vi "Init.vi"(8 "error in (no error)":errorcluster, 11 "XML Report in":refnum<class "Report.lvclass">) -> (0 "error out":errorcluster, 3 "XML Report out":refnum<class "Report.lvclass">)   [LabVIEW 2020, in "Reports.lvlib" / "Report.lvclass"]
uses:
  Report.lvclass
  C:/git/astemes-lunit/source/Framework/Report Interface/Report Interface.lvclass
  Report.lvclass/Report.ctl
  Report Generator/Report Generator.lvclass
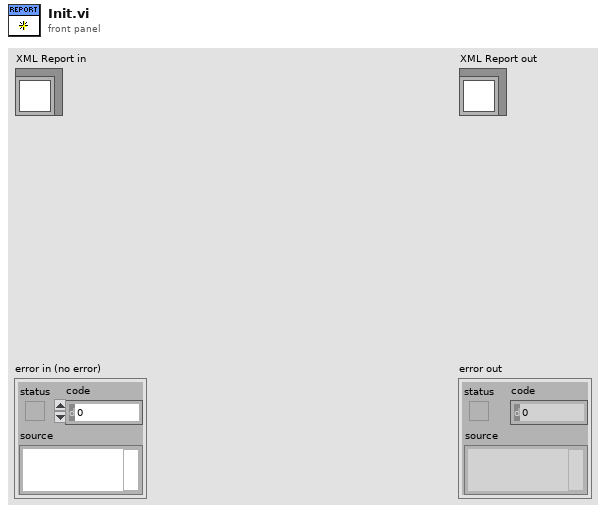
[diagram p1: front panel]
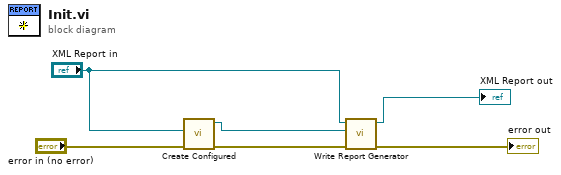
[diagram p0: block diagram]
diagram:
  n1 = call "Create Configured.vi"("error in (no error)"="error in (no error)", "Report Interface"="XML Report in") -> ("error out"=w5:errorcluster, "Report Generator Out"=w2:refnum<class "Report Generator.lvclass">)  [unwired: 8 in]
  n2 = call "Write Report Generator.vi"("error in (no error)"=w5, "Report Generator"=w2, "Report In"="XML Report in") -> ("error out"=→"error out":errorcluster, "Report Out"=→"XML Report out":refnum<class "Report.lvclass">)  [unwired: 7 in]
